vi "as UINT32.vi"(11 "bytes":u8[](array[numeric]) format="%b") -> (3 "UINT32":u32)   [LabVIEW 2020, in "MessagePack.lvlib" / "MessagePackNumeric.lvclass"]
uses:
  MessagePackNumeric.lvclass
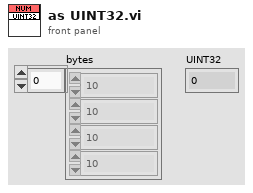
[diagram p1: front panel]
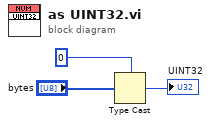
[diagram p0: block diagram]
diagram:
  n1 = Type Cast(type=u32 0 ("INT8"), x="bytes") -> (*(type *) &x=→"UINT32":u32)
